vi "Close.vi"(8 "error in":errorcluster, 11 "TCP in":refnum<class "TCP.lvclass">) -> (0 "error out":errorcluster, 3 "TCP out":refnum<class "TCP.lvclass">)   [LabVIEW 2021, in "TCP.lvclass"]
uses:
  TCP.lvclass
  TCP.lvclass/TCP.ctl
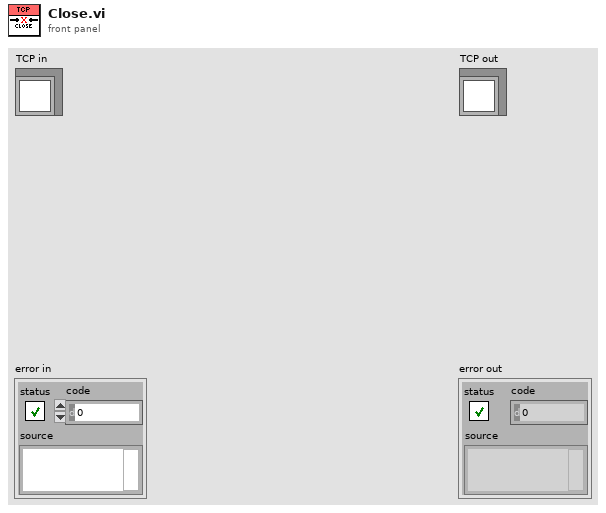
[diagram p1: front panel]
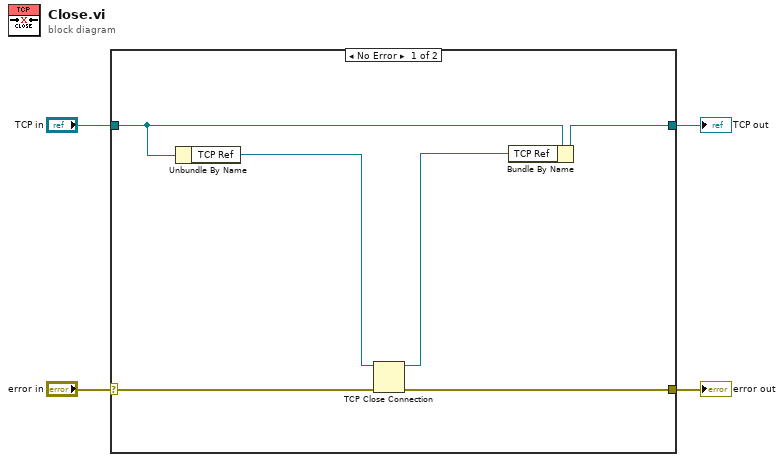
[diagram p0: block diagram]
diagram:
  n1 = case shown="No Error" "error in" {
    selector: "error in" -> [w10 w11]
    tunnel: [w9 w11] -> w3
    tunnel: "TCP in" -> [w8 w12]
    tunnel: [w6 w12] -> w1
    frame No Error {
      n2 = Unbundle By Name(w8) -> ("TCP Ref"=w7:refnum<k5>)
      n3 = TCP Close Connection(connection ID=w7, error in (no error)=w10) -> (connection ID out=w5:refnum<k5>, error out=w9:errorcluster)  [unwired: 1 in]
      n4 = Bundle By Name(cluster=w8, "TCP Ref"=w5) -> (w6:refnum<class "TCP.lvclass">)
    }
    frame Error {
    }
  }
  "error out" <- w3
  "TCP out" <- w1
